vi "APS line.vi"(0 "Dimension":i32, 1 "TransPara":dbl, 5 "Axis_ID_Array":i32[](array[numeric]), 7 "Option":i32, 9 "PositionArray":dbl[](array[numeric]), 11 "error in (no error)":errorcluster caption="错误输入（无错误）", 12 "Wait":cluster{"h_event":u32, "i32_ret":i32}) -> (3 "TransPara out":dbl, 4 "function return":i32, 10 "PositionArray 2":dbl[](array[numeric]), 14 "Wait out":cluster{"h_event":u32, "i32_ret":i32}, 15 "error out":errorcluster caption="错误输出")   [LabVIEW 2011, in "APS168.lvlib"]
doc: "I32 FNTYPE APS_line( I32 Dimension, I32 *Axis_ID_Array, I32 Option, F64 *PositionArray, F64 *TransPara, ASYNCALL *Wait);"
uses:
  APS168.lvlib
panel:
  out "Axis_ID_Array":i32[](array[numeric])
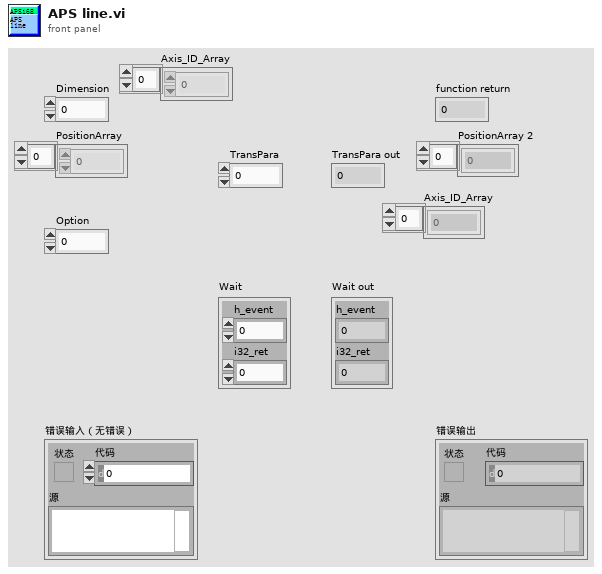
[diagram p1: front panel]
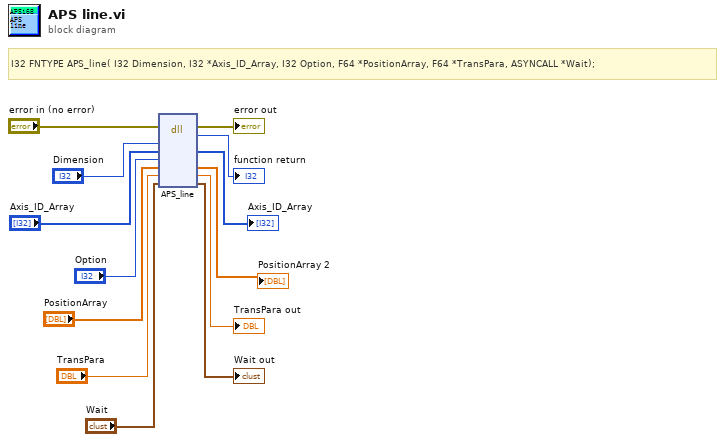
[diagram p0: block diagram]
diagram:
  # "I32 FNTYPE APS_line( I32 Dimension, I32 *Axis_ID_Array, I32 Option, F64 *PositionArray, F64 *TransPara, ASYNCALL *Wait);"
  n1 = dll-call lib="PTH1Labs E软件ADLINK 204CAPS_1_7_1_LIB line 连续运动204APS168.*" fn="APS_line"(error in="error in (no error)", "Dimension"="Dimension", "Axis_ID_Array"="Axis_ID_Array", "Option"="Option", "PositionArray"="PositionArray", "TransPara"="TransPara", "Wait"="Wait") -> (error out=→"error out":errorcluster, "返回类型"=→"function return":i32, "Axis_ID_Array"=→"Axis_ID_Array":i32[], "PositionArray"=→"PositionArray 2":dbl[], "TransPara"=→"TransPara out":dbl, "Wait"=→"Wait out":cluster{"h_event":u32, "i32_ret":i32})  [unwired: 4 in, 1 out]
